vi "display_1s_stim_9s_ISI_CS1_CS2_timeout.vi"() -> ()   [LabVIEW 2019]
uses:
  <vilib>/Analysis/Matrix/Datatypes/RealMatrix.ctl
  <vilib>/Utility/file.llb/Write Delimited Spreadsheet (DBL).vi
  <vilib>/Analysis/Matrix/NI_Matrix.lvlib
panel:
  out "Num trials":u32=204
  out "ISI Time":dbl
  out "Stim TS":dbl
  out "Output":dbl[][](array[numeric])
  out "Output frame":T1
  out "Array temp1":T1
  out "Elapsed Time":dbl
  out "Display":bool=TRUE
  out "Trial":u32=1
  out "reward":dbl[](array[numeric])
  out "stim_id":dbl[](array[numeric])
  out "stim_loaded":dbl
  out "Timings":dbl[](array[numeric])
  out "Stimuli Loaded?":bool
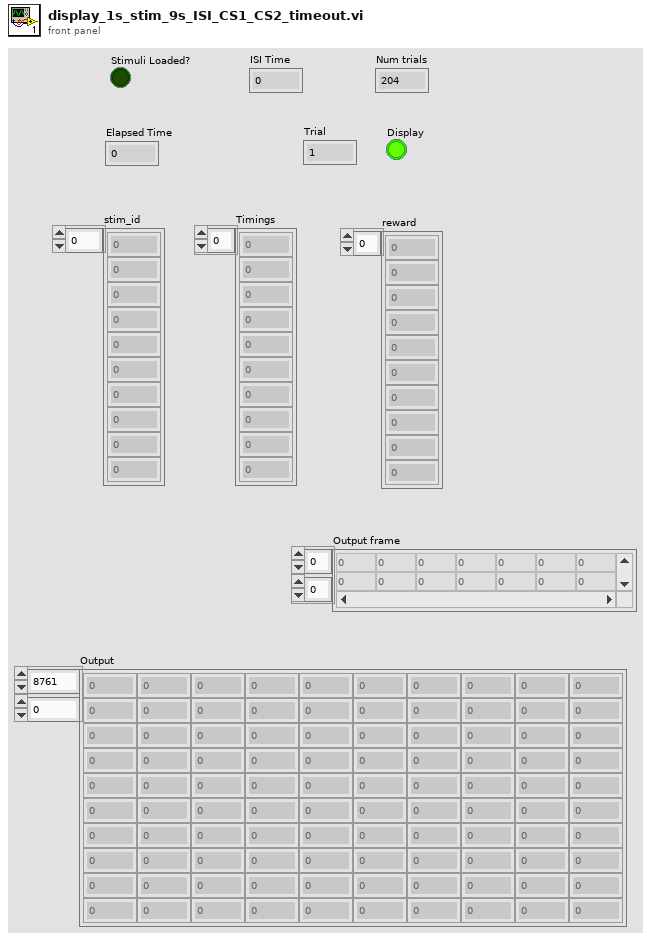
[diagram p1: front panel]
types:
  T1 = typedef "NI_Matrix.lvlib/RealMatrix.ctl" = dbl[][]
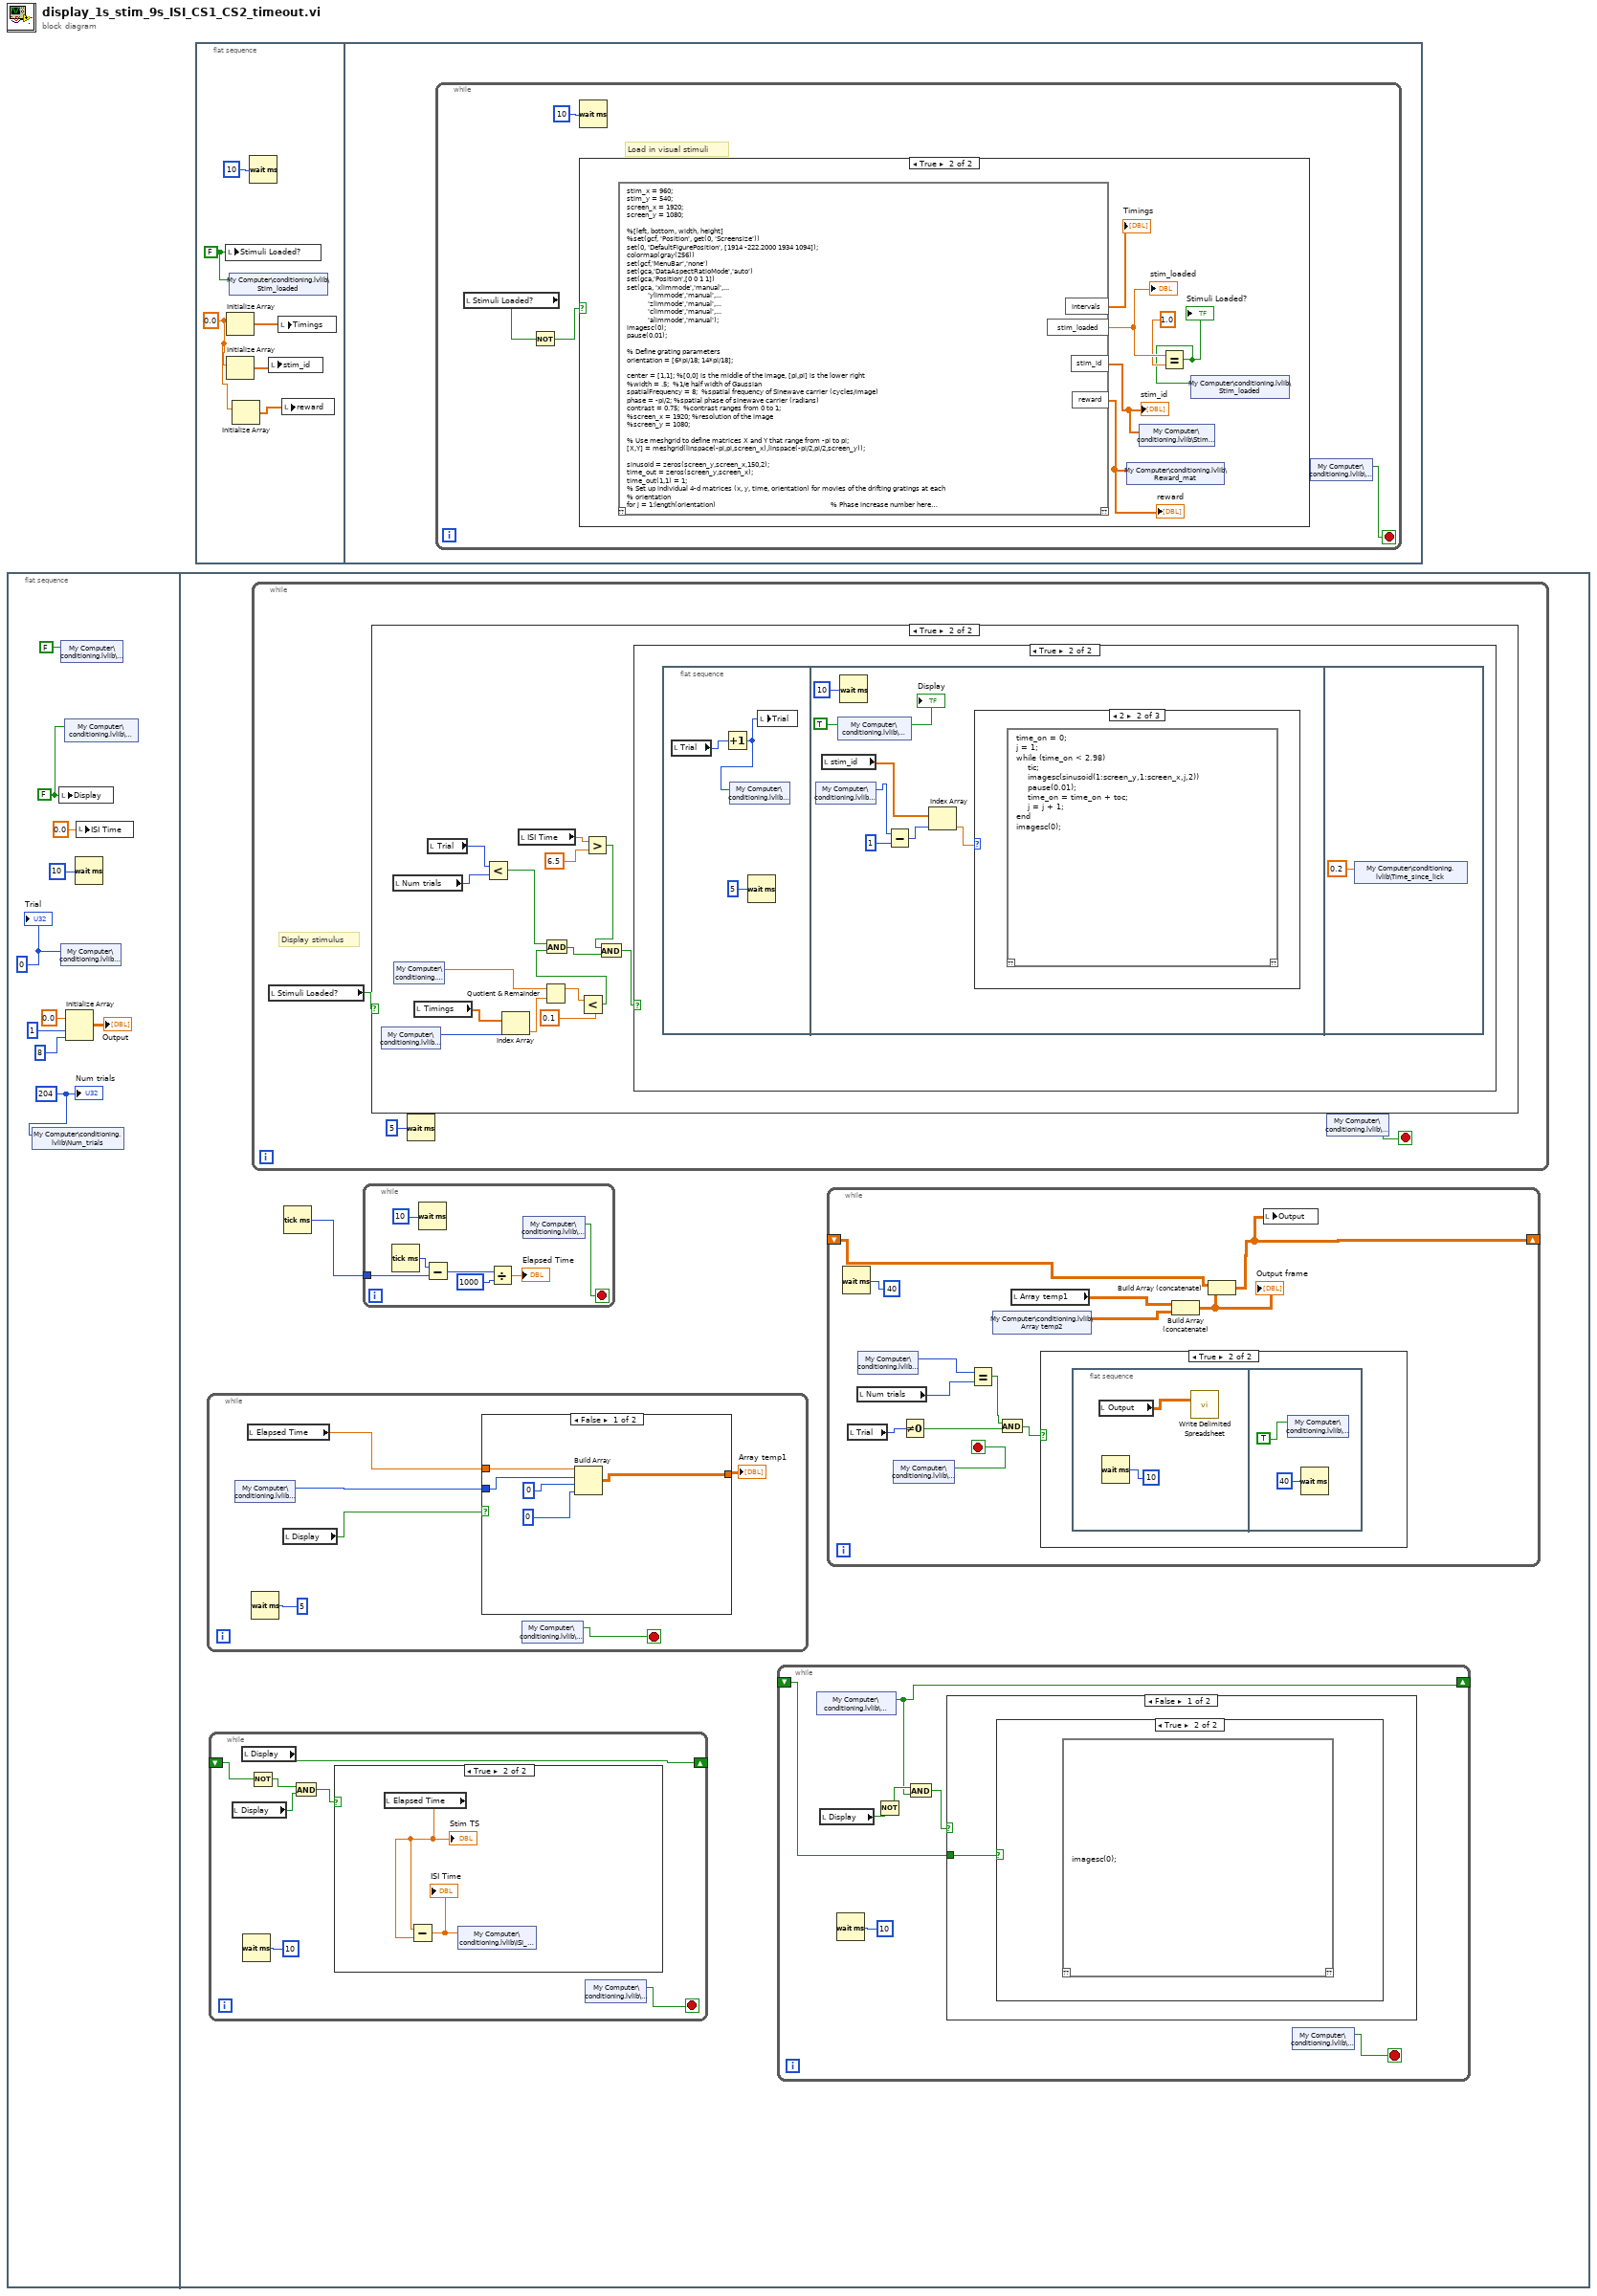
[diagram p0: block diagram]
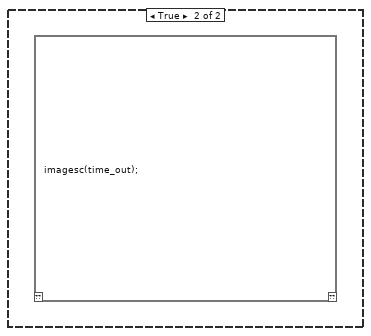
[diagram p4: hidden frame]
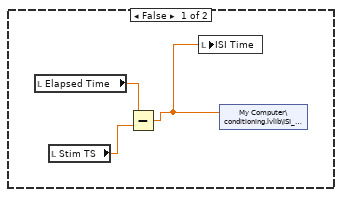
[diagram p5: hidden frame]
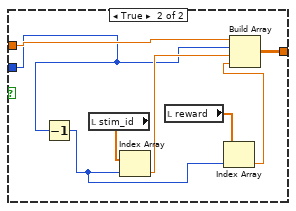
[diagram p6: hidden frame]
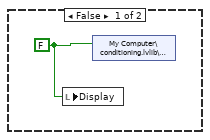
[diagram p9: hidden frame]
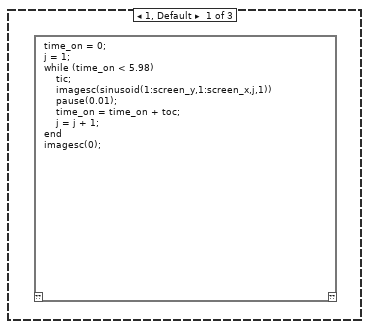
[diagram p10: hidden frame]
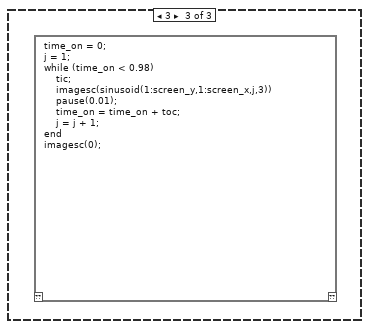
[diagram p11: hidden frame]
diagram:
  n1 = flat-sequence {
    frame #0 {
      w2 = u32 204
      w8 = FALSE ("Display")
      w10 = u32 0 ("Trial")
      n2 = shared-variable "My Computer\\conditioning.lvlib\\Num_trials"(w2) -> ()  [unwired: 1 in, 1 out]
      n3 = local write "Display"(w8) -> ()
      n4 = shared-variable "My Computer\\conditioning.lvlib\\Stop"(FALSE ("Stop")) -> ()  [unwired: 1 in, 1 out]
      n5 = shared-variable "My Computer\\conditioning.lvlib\\Trial"(w10) -> ()  [unwired: 1 in, 1 out]
      n6 = shared-variable "My Computer\\conditioning.lvlib\\Display"(w8) -> ()  [unwired: 1 in, 1 out]
      n7 = Initialize Array(0.0 ("element"), 1 ("dimension size"), 8 ("dimension size")) -> (→"Output":dbl[][])
      n8 = Wait (ms)(milliseconds to wait=u32 10) -> ()  [unwired: 1 out]
      n9 = local write "ISI Time"(0.0 ("ISI Time")) -> ()
      "Trial" <- w10
      "Num trials" <- w2
    }
    frame #1 {
      n10 = while {
        stop <- w32 stop-if-true
        n11 = shared-variable "My Computer\\conditioning.lvlib\\Trial"() -> (w34:u32)  [unwired: 1 in, 1 out]
        n12 = local read "Elapsed Time"() -> (w36:dbl)
        n13 = Wait (ms)(milliseconds to wait=u32 5) -> ()  [unwired: 1 out]
        n14 = local read "Display"() -> (w33:bool)
        n15 = case shown="False" w33 {
          tunnel: w34 -> [w41 w46]
          tunnel: w36 -> [w42 w48]
          tunnel: [w40 w49] -> w35
          frame False {
            n16 = Build Array(w42, w41, u32 0 ("milliseconds to wait"), 0) -> (w40:T1)
          }
          frame True {
            n17 = Decrement(x=w46) -> (x-1=w44:u32)
            n18 = local read "stim_id"() -> (w50:dbl[])
            n19 = Index Array(array=w50, index=w44) -> (element=w47:dbl)
            n20 = local read "reward"() -> (w45:dbl[])
            n21 = Index Array(array=w45, index=w44) -> (element=w43:dbl)
            n22 = Build Array(w48, w46, w47, w43) -> (w49:T1)
          }
        }
        "Array temp1" <- w35
        n23 = shared-variable "My Computer\\conditioning.lvlib\\Stop"() -> (w32:bool)  [unwired: 1 in, 1 out]
      }
      n24 = while {
        shift-right: [w24] -> _
        shift-left: _ -> [w23]
        stop <- w26 stop-if-true
        n25 = local read "Display"() -> (w21:bool)
        n26 = local read "Display"() -> (w24:bool)
        n27 = Wait (ms)(milliseconds to wait=u32 10) -> ()  [unwired: 1 out]
        n28 = Not(x=w23) -> (.not. x?=w22:bool)
        n29 = And(x=w22, y=w21) -> (x .and. y?=w20:bool)
        n30 = case shown="True" w20 {
          frame False {
            n31 = local read "Elapsed Time"() -> (w27:dbl)
            n32 = local read "Stim TS"() -> (w29:dbl)
            n33 = Subtract(x=w27, y=w29) -> (x-y=w28:dbl)
            n34 = local write "ISI Time"(w28) -> ()
            n35 = shared-variable "My Computer\\conditioning.lvlib\\ISI_Time"(w28) -> ()  [unwired: 1 in, 1 out]
          }
          frame True {
            n36 = local read "Elapsed Time"() -> (w30:dbl)
            "Stim TS" <- w30
            n37 = Subtract(x=w30, y=w30) -> (x-y=w31:dbl)
            "ISI Time" <- w31
            n38 = shared-variable "My Computer\\conditioning.lvlib\\ISI_Time"(w31) -> ()  [unwired: 1 in, 1 out]
          }
        }
        n39 = shared-variable "My Computer\\conditioning.lvlib\\Stop"() -> (w26:bool)  [unwired: 1 in, 1 out]
      }
      n40 = while {
        stop <- w76 stop-if-true
        # "Display stimulus"
        n41 = local read "Stimuli Loaded?"() -> (w75:bool)
        n42 = case shown="True" w75 {
          frame False {
          }
          frame True {
            n43 = shared-variable "My Computer\\conditioning.lvlib\\Trial"() -> (w85:u32)  [unwired: 1 in, 1 out]
            n44 = local read "Num trials"() -> (w84:u32)
            n45 = shared-variable "My Computer\\conditioning.lvlib\\ISI"() -> (w83:dbl)  [unwired: 1 in, 1 out]
            n46 = local read "Timings"() -> (w90:dbl[])
            n47 = local read "Trial"() -> (w88:u32)
            n48 = Less?(x=w88, y=w84) -> (x < y?=w87:bool)
            n49 = Index Array(array=w90, index=w85) -> (element=w89:dbl)
            n50 = local read "ISI Time"() -> (w81:dbl)
            n51 = Quotient & Remainder(x=w83, y=w89) -> (x-y*floor(x/y)=w92:dbl)  [unwired: 1 out]
            n52 = Less?(x=w92, y=0.1) -> (x < y?=w86:bool)
            n53 = And(x=w87, y=w86) -> (x .and. y?=w82:bool)
            n54 = Greater?(x=w81, y=6.5) -> (0:w79:bool)
            n55 = And(x=w79, y=w82) -> (x .and. y?=w78:bool)
            n56 = case shown="True" w78 {
              frame False {
                w93 = FALSE ("Display")
                n57 = local write "Display"(w93) -> ()
                n58 = shared-variable "My Computer\\conditioning.lvlib\\Display"(w93) -> ()  [unwired: 1 in, 1 out]
              }
              frame True {
                n59 = flat-sequence {
                  frame #0 {
                    n60 = local read "Trial"() -> (w95:u32)
                    n61 = Increment(x=w95) -> (x+1=w94:u32)
                    n62 = shared-variable "My Computer\\conditioning.lvlib\\Trial"(w94) -> ()  [unwired: 1 in, 1 out]
                    n63 = Wait (ms)(milliseconds to wait=u32 5) -> ()  [unwired: 1 out]
                    n64 = local write "Trial"(w94) -> ()
                  }
                  frame #1 {
                    w101 = TRUE ("Boolean")
                    n65 = shared-variable "My Computer\\conditioning.lvlib\\Trial"() -> (w99:u32)  [unwired: 1 in, 1 out]
                    n66 = local read "stim_id"() -> (w102:dbl[])
                    n67 = shared-variable "My Computer\\conditioning.lvlib\\Display"(w101) -> ()  [unwired: 1 in, 1 out]
                    n68 = Wait (ms)(milliseconds to wait=u32 10) -> ()  [unwired: 1 out]
                    n69 = Subtract(x=w99, y=u32 1) -> (x-y=w100:u32)
                    n70 = Index Array(array=w102, index=w100) -> (element=w97:dbl)
                    n71 = case shown="2" w97 {
                      frame 1, Default {
                        n72 = script code="time_on = 0;\nj = 1;\nwhile (time_on < 5.98)\n    tic;\n    imagesc(sinusoid(1:screen_y,1:screen_x,j,1))\n    pause(0.01);\n    time_on = time_on + toc;\n    j = j + 1;\nend\nimagesc(0);"() -> ()  [unwired: 1 in, 1 out]
                      }
                      frame 2 {
                        n73 = script code="time_on = 0;\nj = 1;\nwhile (time_on < 2.98)\n    tic;\n    imagesc(sinusoid(1:screen_y,1:screen_x,j,2))\n    pause(0.01);\n    time_on = time_on + toc;\n    j = j + 1;\nend\nimagesc(0);"() -> ()  [unwired: 1 in, 1 out]
                      }
                      frame 3 {
                        n74 = script code="time_on = 0;\nj = 1;\nwhile (time_on < 0.98)\n    tic;\n    imagesc(sinusoid(1:screen_y,1:screen_x,j,3))\n    pause(0.01);\n    time_on = time_on + toc;\n    j = j + 1;\nend\nimagesc(0);"() -> ()  [unwired: 1 in, 1 out]
                      }
                    }
                    "Display" <- w101
                  }
                  frame #2 {
                    n75 = shared-variable "My Computer\\conditioning.lvlib\\Time_since_lick"(0.2 ("Time_since_lick")) -> ()  [unwired: 1 in, 1 out]
                  }
                }
              }
            }
          }
        }
        n76 = Wait (ms)(milliseconds to wait=u32 5) -> ()  [unwired: 1 out]
        n77 = shared-variable "My Computer\\conditioning.lvlib\\Stop"() -> (w76:bool)  [unwired: 1 in, 1 out]
      }
      n78 = Tick Count (ms)() -> (millisecond timer value=w11:u32)
      n79 = while {
        tunnel: w11 -> [w54]
        stop <- w51 stop-if-true
        n80 = Tick Count (ms)() -> (millisecond timer value=w55:u32)
        n81 = Wait (ms)(milliseconds to wait=u32 10) -> ()  [unwired: 1 out]
        n82 = Subtract(x=w55, y=w54) -> (x-y=w52:u32)
        n83 = Divide(x=w52, y=u32 1000) -> (x/y=→"Elapsed Time":dbl)
        n84 = shared-variable "My Computer\\conditioning.lvlib\\Stop"() -> (w51:bool)  [unwired: 1 in, 1 out]
      }
      n85 = while {
        shift-right: [w13] -> _
        shift-left: _ -> [w12]
        stop <- w18 stop-if-true
        n86 = shared-variable "My Computer\\conditioning.lvlib\\Timeout"() -> (w13:bool)  [unwired: 1 in, 1 out]
        n87 = local read "Display"() -> (w15:bool)
        n88 = Wait (ms)(milliseconds to wait=u32 10) -> ()  [unwired: 1 out]
        n89 = Not(x=w15) -> (.not. x?=w16:bool)
        n90 = And(x=w16, y=w13) -> (x .and. y?=w14:bool)
        n91 = case shown="False" w14 {
          tunnel: w12 -> [w19 _]
          frame False {
            n92 = case shown="True" w19 {
              frame False {
              }
              frame True {
                n93 = script code="imagesc(0);"() -> ()  [unwired: 1 in, 1 out]
              }
            }
          }
          frame True {
            n94 = script code="imagesc(time_out);"() -> ()  [unwired: 1 in, 1 out]
          }
        }
        n95 = shared-variable "My Computer\\conditioning.lvlib\\Stop"() -> (w18:bool)  [unwired: 1 in, 1 out]
      }
      n96 = while {
        shift-right: [w67] -> _
        shift-left: _ -> [w68]
        stop <- w70 stop-if-true
        n97 = Wait (ms)(milliseconds to wait=u32 40) -> ()  [unwired: 1 out]
        n98 = local read "Trial"() -> (w60:u32)
        n99 = local read "Num trials"() -> (w62:u32)
        n100 = shared-variable "My Computer\\conditioning.lvlib\\Trial"() -> (w63:u32)  [unwired: 1 in, 1 out]
        n101 = shared-variable "My Computer\\conditioning.lvlib\\Stop"() -> (w70:bool)  [unwired: 1 in, 1 out]
        n102 = Not Equal To 0?(x=w60) -> (x != 0?=w59:bool)
        n103 = Equal?(x=w63, y=w62) -> (x = y?=w61:bool)
        n104 = shared-variable "My Computer\\conditioning.lvlib\\Array temp2"() -> (w65:dbl[][])  [unwired: 1 in, 1 out]
        n105 = And(x=w61, y=w59) -> (x .and. y?=w58:bool)
        n106 = local read "Array temp1"() -> (w66:T1)
        n107 = case shown="True" w58 {
          frame False {
          }
          frame True {
            n108 = flat-sequence {
              frame #0 {
                n109 = local read "Output"() -> (w72:dbl[][])
                n110 = Wait (ms)(milliseconds to wait=u32 10) -> ()  [unwired: 1 out]
                n111 = call-poly <vilib>:"Write Delimited Spreadsheet.vi"("2D data"=w72) -> ()  [unwired: 13 in, 2 out]
              }
              frame #1 {
                n112 = shared-variable "My Computer\\conditioning.lvlib\\Stop"(TRUE) -> ()  [unwired: 1 in, 1 out]
                n113 = Wait (ms)(milliseconds to wait=u32 40) -> ()  [unwired: 1 out]
              }
            }
          }
        }
        n114 = Build Array (concatenate)(w66, w65) -> (w64:T1)
        "Output frame" <- w64
        n115 = Build Array (concatenate) ("Build Matrix")(w68, w64) -> (w67:T1)
        n116 = local write "Output"(w67) -> ()
      }
    }
  }
  n117 = flat-sequence {
    frame #0 {
      w107 = 0.0 ("element")
      w105 = FALSE ("Stimuli Loaded?")
      n118 = local write "Stimuli Loaded?"(w105) -> ()
      n119 = Initialize Array(w107) -> (w109:dbl[])  [unwired: 1 in]
      n120 = Initialize Array(w107) -> (w108:dbl[])  [unwired: 1 in]
      n121 = shared-variable "My Computer\\conditioning.lvlib\\Stim_loaded"(w105) -> ()  [unwired: 1 in, 1 out]
      n122 = Initialize Array(w107) -> (w106:dbl[])  [unwired: 1 in]
      n123 = Wait (ms)(milliseconds to wait=u32 10) -> ()  [unwired: 1 out]
      n124 = local write "stim_id"(w108) -> ()
      n125 = local write "Timings"(w109) -> ()
      n126 = local write "reward"(w106) -> ()
    }
    frame #1 {
      n127 = while {
        stop <- w113 stop-if-true
        # "Load in visual stimuli"
        n128 = local read "Stimuli Loaded?"() -> (w112:bool)
        n129 = Not(x=w112) -> (.not. x?=w111:bool)
        n130 = Wait (ms)(milliseconds to wait=u32 10) -> ()  [unwired: 1 out]
        n131 = case shown="True" w111 {
          frame False {
          }
          frame True {
            n132 = script code="stim_x = 960;\nstim_y = 540;\nscreen_x = 1920;\nscreen_y = 1080;\n\n%[left, bottom, width, height]\n%set(gcf, 'Position', get(0, 'Screensize'))\nset(0, 'DefaultFigurePosition', [1914 -222.2000 1934 1094]);\ncolormap(gray(256))\nset(gcf,'MenuBar','none')\nset(gca,'DataAspectRatioMode','auto')\nset(gca,'Position',[0 0 1 1])\nset(gca, 'xlimmode','manual',...\n           'ylimmode','manual',...\n           'zlimmode','manual',...\n           'climmode','manual',...\n           'alimmode','manual');\nimagesc(0);\npause(0.01);\n\n% Define grating parameters\norientation = [6*pi/18; 14*pi/18];\n\ncenter = [1,1]; %[0,0] is the middle of the image, [pi,pi] is the lower right\n%width = .5;  %1/e half width of Gaussian\nspatialFrequency = 8;  %spatial frequency of Sinewave carrier (cycles/image)\nphase = -pi/2; %spatial phase of sinewave carrier (radians)\ncontrast = 0.75;  %contrast ranges from 0 to 1;\n%screen_x = 1920; %resolution of the image  \n%screen_y = 1080;\n\n% Use meshgrid to define matrices X and Y that range from -pi to pi;\n[X,Y] = meshgrid(linspace(-pi,pi,screen_x),linspace(-pi/2,pi/2,screen_y));\n\nsinusoid = zeros(screen_y,screen_x,150,2);\ntime_out = zeros(screen_y,screen_x);\ntime_out(1,1) = 1;\n% Set up individual 4-d matrices (x, y, time, orientation) for movies of the drifting gratings at each\n% orientation\nfor j = 1:length(orientation)                                                            % Phase increase number here\n    ramp(1:screen_y,1:screen_x,j) = cos(orientation(j))*(X-center(1)) + sin(orientation(j))*(Y-center(2));     %  |\n    for i = 1:150 %Sets the number of frames to define gratings for                   V\n       sinusoid(1:screen_y,1:screen_x,i,j) = contrast*sin(spatialFrequency*ramp(1:screen_y,1:screen_x,j)-...\n           (phase+(2*pi*(i-1)*(-30)/360))); %Number before '/360' sets the phase increase\n    end\nend\n\n%intervals = [ones(1,41)*10 ones(1,41)*11 ones(1,41)*12 ones(1,41)*13 ones(1,40)*14];\nintervals = [ones(1,204)*3];\nintervals = intervals(randperm(204));\nrand_idx1 = randperm(204);\nrand_idx2 = randperm(204);\nstim_id = [ones(1,102)*1 ones(1,102)*2];\n%reward = [ones(1,87)*1 ones(1,15)*0 ones(1,87)*1 ones(1,15)*0];\nreward = [ones(1,204)*1];\nstim_id = stim_id(rand_idx2);\nreward = reward(rand_idx2);\n\nstim_loaded = 1;" ("Script Node")() -> ("stim_loaded"=w120:dbl, "intervals"=→"Timings":dbl[], "stim_id"=w115:dbl[], "reward"=w117:dbl[])  [unwired: 1 in, 1 out]
            "stim_loaded" <- w120
            "stim_id" <- w115
            "reward" <- w117
            n133 = shared-variable "My Computer\\conditioning.lvlib\\Reward_mat"(w117) -> ()  [unwired: 1 in, 1 out]
            n134 = shared-variable "My Computer\\conditioning.lvlib\\Stim_ID"(w115) -> ()  [unwired: 1 in, 1 out]
            n135 = Equal?(x=w120, y=1.0) -> (x = y?=w116:bool)
            "Stimuli Loaded?" <- w116
            n136 = shared-variable "My Computer\\conditioning.lvlib\\Stim_loaded"(w116) -> ()  [unwired: 1 in, 1 out]
          }
        }
        n137 = shared-variable "My Computer\\conditioning.lvlib\\Stop"() -> (w113:bool)  [unwired: 1 in, 1 out]
      }
    }
  }
